vi "publish status.vi"(8 "error in (no error)":errorcluster, 11 "Channel in":refnum<class "Channel.lvclass">) -> (0 "error out":errorcluster, 3 "Channel out":refnum<class "Channel.lvclass">)   [LabVIEW 2018, in "Channel.lvclass"]
uses:
  Channel.lvclass
  Channel.lvclass/Channel.ctl
  State Machine/State Machine.lvclass/State Machine.ctl
  State Machine/State Machine.lvclass
  Simulated_CCD_Camera/Simulated Camera.lvclass
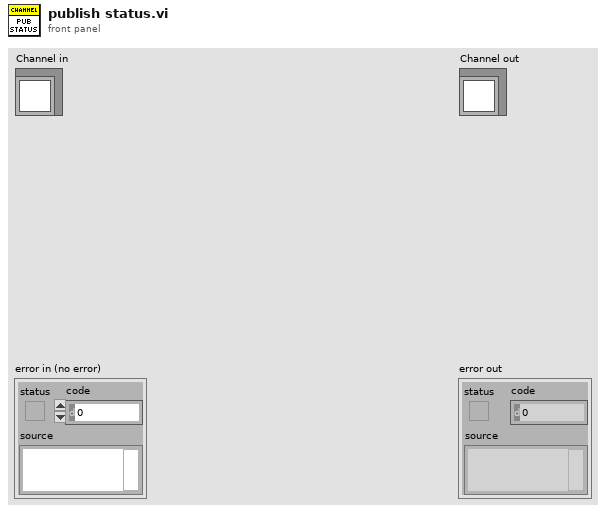
[diagram p1: front panel]
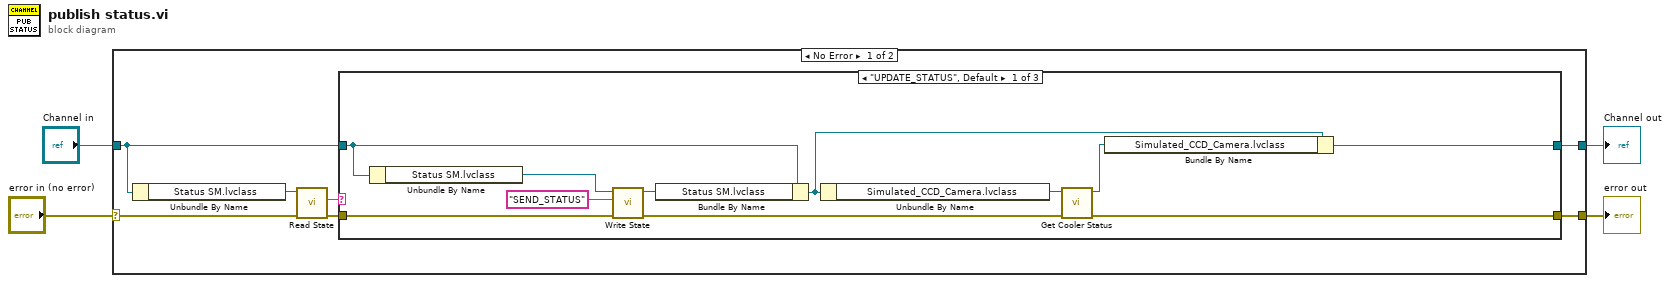
[diagram p0: block diagram]
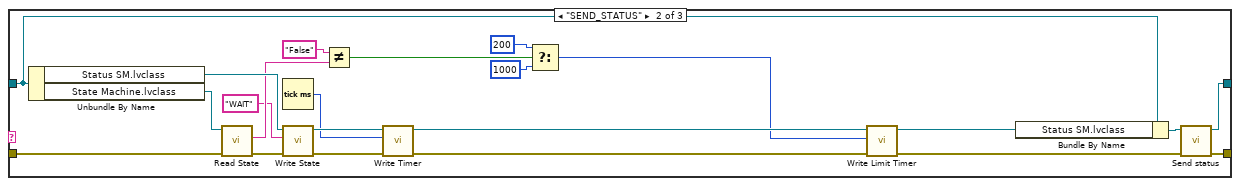
[diagram p2: hidden frame]
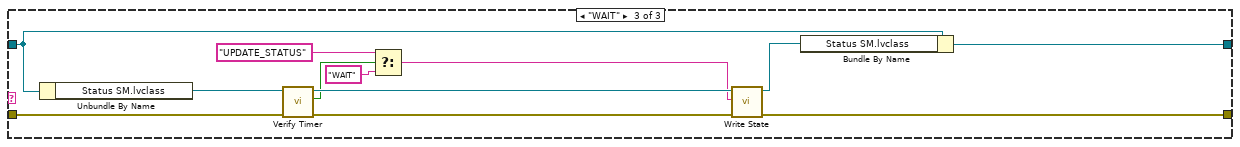
[diagram p3: hidden frame]
diagram:
  n1 = case shown="No Error" "error in (no error)" {
    selector: "error in (no error)" -> [w10 w58]
    tunnel: [w5 w58] -> w3
    tunnel: [w7 w57] -> w1
    tunnel: "Channel in" -> [w6 w57]
    frame No Error {
      n2 = Unbundle By Name(w6) -> ("Status SM.lvclass"=w11:refnum<class "State Machine.lvclass">)
      n3 = call-dynamic "Read State.vi"("error in (no error)"=w10, "State Machine in"=w11) -> ("error out"=w8:errorcluster, "State"=w9:string)  [unwired: 7 in, 1 out]
      n4 = case shown="\"UPDATE_STATUS\", Default" w9 {
        tunnel: w6 -> [w17 w28 w55]
        tunnel: w8 -> [w18 w29 w56]
        tunnel: [w14 w24 w49] -> w5
        tunnel: [w16 w23 w53] -> w7
        frame "UPDATE_STATUS", Default {
          n5 = Unbundle By Name(w17) -> ("Status SM.lvclass"=w20:refnum<class "State Machine.lvclass">)
          n6 = call-dynamic "Write State.vi"("error in (no error)"=w18, "State"="SEND_STATUS", "State Machine in"=w20) -> ("error out"=w12:errorcluster, "State Machine out"=w21:refnum<class "State Machine.lvclass">)  [unwired: 7 in]
          n7 = Bundle By Name(cluster=w17, "Status SM.lvclass"=w21) -> (w22:refnum<class "Channel.lvclass">)
          n8 = Unbundle By Name(w22) -> ("Simulated_CCD_Camera.lvclass"=w13:refnum<class "Simulated Camera.lvclass">)
          n9 = call-dynamic "Get Cooler Status.vi"("error in (no error)"=w12, "CCDCamera in"=w13) -> ("error out"=w14:errorcluster, "CCDCamera out"=w15:refnum<class "Simulated Camera.lvclass">)  [unwired: 8 in]
          n10 = Bundle By Name(cluster=w22, "Simulated_CCD_Camera.lvclass"=w15) -> (w16:refnum<class "Channel.lvclass">)
        }
        frame "SEND_STATUS" {
          n11 = Unbundle By Name(w28) -> ("Status SM.lvclass"=w37:refnum<class "State Machine.lvclass">, "State Machine.lvclass"=w38:refnum<class "State Machine.lvclass">)
          n12 = call-dynamic "Read State.vi"("error in (no error)"=w29, "State Machine in"=w38) -> ("error out"=w36:errorcluster, "State"=w35:string)  [unwired: 7 in, 1 out]
          n13 = Tick Count (ms)() -> (millisecond timer value=w42:u32)
          n14 = call-dynamic "Write State.vi"("error in (no error)"=w36, "State"="WAIT", "State Machine in"=w37) -> ("error out"=w43:errorcluster, "State Machine out"=w44:refnum<class "State Machine.lvclass">)  [unwired: 7 in]
          n15 = Not Equal?(x="False" ("State"), y=w35) -> (x != y?=w27:bool)
          n16 = call "Write Timer.vi"("error in (no error)"=w43, "Timer"=w42, "State Machine in"=w44) -> ("error out"=w39:errorcluster, "State Machine out"=w41:refnum<class "State Machine.lvclass">)  [unwired: 7 in]
          n17 = Select(t=200, s=w27, f=1000) -> (s? t:f=w34:i32)
          n18 = call "Write Limit Timer.vi"("error in (no error)"=w39, "Limit Timer"=w34, "State Machine in"=w41) -> ("error out"=w25:errorcluster, "State Machine out"=w40:refnum<class "State Machine.lvclass">)  [unwired: 7 in]
          n19 = Bundle By Name(cluster=w28, "Status SM.lvclass"=w40) -> (w26:refnum<class "Channel.lvclass">)
          n20 = call "Send status.vi"("error in (no error)"=w25, "Channel in"=w26) -> ("error out"=w24:errorcluster, "Channel out"=w23:refnum<class "Channel.lvclass">)  [unwired: 8 in]
        }
        frame "WAIT" {
          n21 = Unbundle By Name(w55) -> ("Status SM.lvclass"=w54:refnum<class "State Machine.lvclass">)
          n22 = call "Verify Timer.vi"("error in (no error)"=w56, "State Machine in"=w54) -> ("error out"=w52:errorcluster, "time out"=w45:bool, "State Machine out"=w51:refnum<class "State Machine.lvclass">)  [unwired: 7 in]
          n23 = Select(t="UPDATE_STATUS", s=w45, f="WAIT") -> (s? t:f=w48:string)
          n24 = call-dynamic "Write State.vi"("error in (no error)"=w52, "State"=w48, "State Machine in"=w51) -> ("error out"=w49:errorcluster, "State Machine out"=w50:refnum<class "State Machine.lvclass">)  [unwired: 7 in]
          n25 = Bundle By Name(cluster=w55, "Status SM.lvclass"=w50) -> (w53:refnum<class "Channel.lvclass">)
        }
      }
    }
    frame Error {
    }
  }
  "error out" <- w3
  "Channel out" <- w1
